vi "_CSMObj-ObtainCore.vi"(7 "Allowed Messages(Empty for all)":string[](array[string]), 8 "Error in":errorcluster caption="Error in (no error)", 11 "Requested Name":string) -> (0 "Error out":errorcluster, 3 "CSMQ out":T1={"Core"={"Module Name"="", "Requested Name"="", "Group Name"="", "Mode"=enum."Stand Alone", "User Event"=refnum, "CSM-Data"=refnum, "Allowed Messages"=[], "WatchDogQ"=refnum}, "Shared"={"Queue"=refnum, "Status Change Event"=refnum, "TagMap"=refnum, "Mode-Data"=refnum, "Exit Event"=refnum}})   [LabVIEW 2017, in "Communicable State Machine.lvlib"]
uses:
  Communicable State Machine.lvlib
  _CSMObj.ctl
  Priority Queue/Priority Queue.lvclass
  Typedef/_CSM_MODE.ctl
  _CSMObj-Data.ctl
  Typedef/_CSM Status Change Event Data.ctl
  _CSMObj-ModeData.ctl
  _Shared/CSM Shared.lvlib
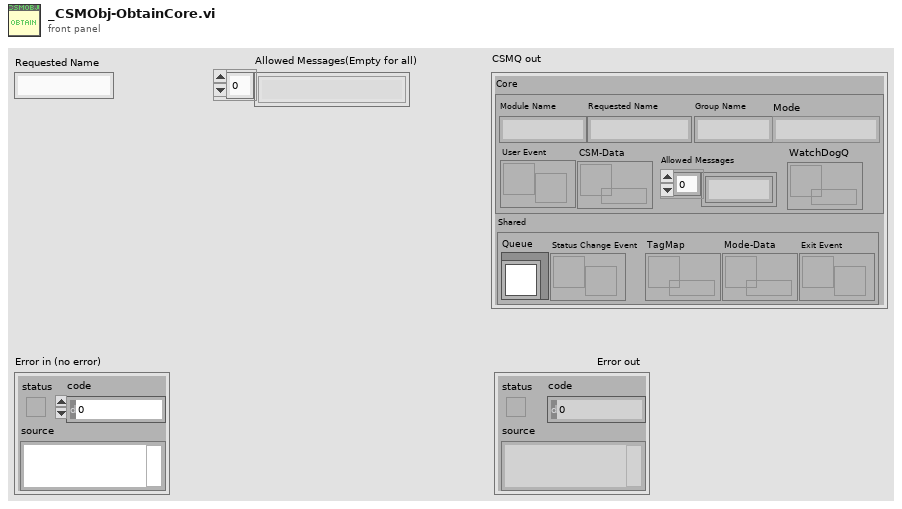
[diagram p1: front panel]
types:
  T1 = typedef "Communicable State Machine.lvlib/_CSMObj.ctl" = cluster{"Core":cluster{"Module Name":string, "Requested Name":string, "Group Name":string, "Mode":T2, "User Event":refnum<user-event>, "CSM-Data":refnum<data-value>, "Allowed Messages":string[], "WatchDogQ":refnum<queue>}, "Shared":cluster{"Queue":refnum<class "Priority Queue.lvclass">, "Status Change Event":refnum<user-event>, "TagMap":refnum<data-value>, "Mode-Data":refnum<data-value>, "Exit Event":refnum<user-event>}}
  T2 = typedef "Communicable State Machine.lvlib/_CSM_MODE.ctl" = enum16{"Not Exist", "Stand Alone", "CSM", "Worker", "Worker Agent", "Chain Node", "Chain"}
  T3 = typedef "Communicable State Machine.lvlib/_CSMObj-Data.ctl" = cluster{"RemoteMessge?":bool, "error":errorcluster, "InternalRegistryRules":string[], "Return State":string}
  T4 = typedef "Communicable State Machine.lvlib/_CSM_NAME_REQUEST.ctl" = enum16{"Stand Alone CSM Request", "Normal CSM Request", "Agent Request", "Action Worker Request", "Chain Request", "Chain Node Request"}
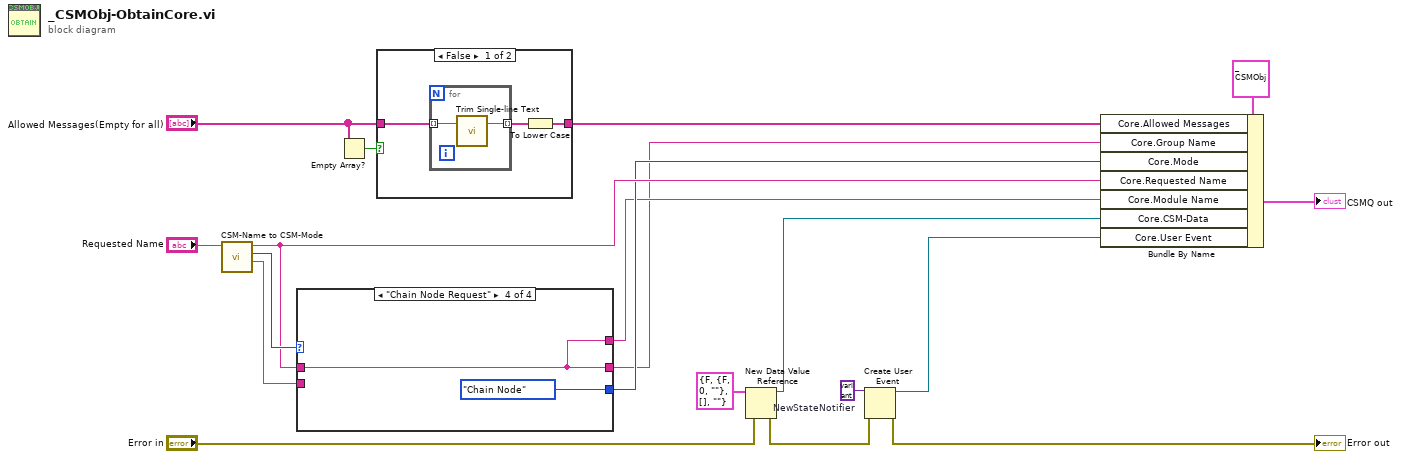
[diagram p0: block diagram]
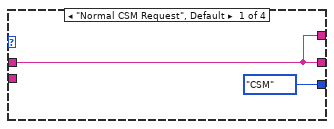
[diagram p2: hidden frame]
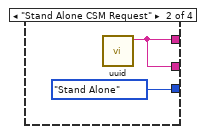
[diagram p3: hidden frame]
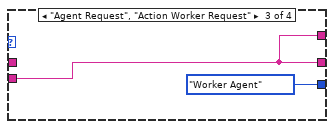
[diagram p4: hidden frame]
diagram:
  w18 = variant  # NewStateNotifier
  n1 = call "CSM-Name to CSM-Mode.vi"("String"="Requested Name") -> ("ParentCSM Name"=w9:string, "CSM Mode"=w7:T4, "Requested Name"=w6:string)  [unwired: 8 in]
  n2 = case shown="\"Chain Node Request\"" w7 {
    tunnel: [w20 w22 w24 w26] -> w2
    tunnel: w6 -> [w20 _ _ w26]
    tunnel: w9 -> [_ _ w24 _]
    tunnel: [_CSM_MODE."CSM" ("Mode") _CSM_MODE."Stand Alone" ("Mode") _CSM_MODE."Worker Agent" ("Mode") _CSM_MODE."Chain Node" ("Mode")] -> w5
    tunnel: [w20 w22 w24 w26] -> w4
    frame "Normal CSM Request", Default {
    }
    frame "Stand Alone CSM Request" {
      n3 = call "uuid.vi"() -> ("UUID"=w22:string)  [unwired: 11 in]
    }
    frame "Agent Request", "Action Worker Request" {
    }
    frame "Chain Node Request" {
    }
  }
  n4 = Empty Array?(array="Allowed Messages(Empty for all)") -> (empty?=w10:bool)
  n5 = case shown="False" w10 {
    tunnel: [w28 w33] -> w12
    tunnel: "Allowed Messages(Empty for all)" -> [w29 w33]
    frame False {
      n6 = for {
        tunnel: [w31] -> w30 mode=indexing
        tunnel: w29 -> [w32] mode=indexing
        n7 = call "Trim Single-line Text.vi"("single-line text"=w32) -> ("trimed text"=w31:string)  [unwired: 2 in]
      }
      n8 = To Lower Case(string=w30) -> (all lower case string=w28:string[])
    }
    frame True {
    }
  }
  n9 = New Data Value Reference(data value=T3 {"RemoteMessge?"=FALSE, "error"={"status"=FALSE, "code"=0, "source"=""}, "InternalRegistryRules"=[], "Return State"=""} ("CSMObj-Data"), error in="Error in") -> (data value reference=w19:refnum<data-value>, error out=w17:errorcluster)
  n10 = Create User Event(user event datatype=w18, error in=w17) -> (user event=w16:refnum<user-event>, error out=→"Error out":errorcluster)
  n11 = Bundle By Name(cluster=T1 {"Core"={"Module Name"="", "Requested Name"="", "Group Name"="", "Mode"=enum."Stand Alone", "User Event"=refnum, "CSM-Data"=refnum, "Allowed Messages"=[], "WatchDogQ"=refnum}, "Shared"={"Queue"=refnum, "Status Change Event"=refnum, "TagMap"=refnum, "Mode-Data"=refnum, "Exit Event"=refnum}} ("CSMQ in"), "Core.Allowed Messages"=w12, "Core.Group Name"=w2, "Core.Mode"=w5, "Core.Requested Name"=w6, "Core.Module Name"=w4, "Core.CSM-Data"=w19, "Core.User Event"=w16) -> (→"CSMQ out":T1)
